vi "HAL process.vi"   [LabVIEW 2016]
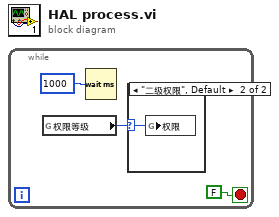
[diagram p0: block diagram]
diagram:
  n1 = while {
    stop <- FALSE stop-if-true
    n2 = global read "非断电保持全局变量.vi" "权限等级"() -> (w2:enum16{"一级权限", "二级权限", "三级权限", "超级权限"})
    n3 = Wait (ms)(milliseconds to wait=u32 1000 ("等待时间（毫秒）")) -> ()  [unwired: 1 out]
    n4 = case shown="\"二级权限\", Default" w2 {
      selector: w2 -> [_ w4]
      frame "一级权限" {
      }
      frame "二级权限", Default {
        n5 = global write "多参数全局变量.vi" "权限"(w4) -> ()
      }
    }
  }
